vi "CRYAddStep Popup Menu.vi"(9 "Tag":string, 10 "Tree Reference In":refnum<vi>, 11 "Menu Ref In":refnum<k9>) -> (3 "Menu Ref Out":refnum<k9>)   [LabVIEW 2013]
uses:
  CRYMainGlobal.vi
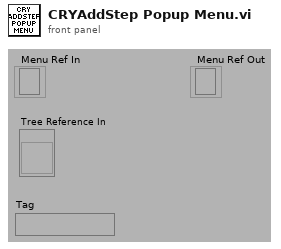
[diagram p1: front panel]
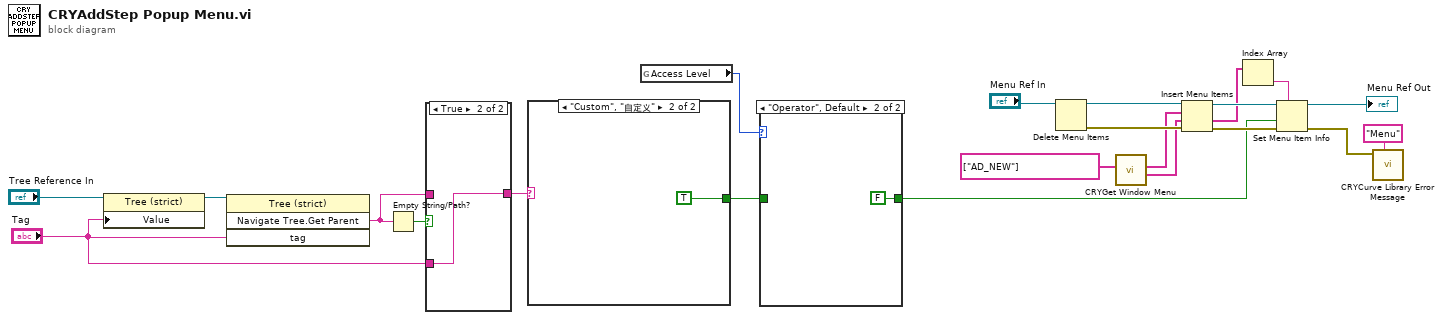
[diagram p0: block diagram]
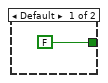
[diagram p3: hidden frame]
diagram:
  n1 = property class="Tree (strict)"(reference="Tree Reference In", "Value"="Tag") -> (reference out=w3:refnum<vi>)  [unwired: 1 in, 1 out]
  n2 = invoke class="Tree (strict)" method="Navigate Tree.Get Parent"(reference=w3, "tag"="Tag") -> ("Navigate Tree:Get Parent"=w15:string)  [unwired: 2 in, 3 out]
  n3 = Empty String/Path?(string/path=w15) -> (empty?=w16:bool)
  n4 = case shown="True" w16 {
    tunnel: w15 -> [w23 _]
    tunnel: [w23 w24] -> w14
    tunnel: "Tag" -> [_ w24]
    frame False {
    }
    frame True {
    }
  }
  n5 = case shown="\"Custom\", \"自定义\"" w14 {
    tunnel: [FALSE ("checked") TRUE ("checked")] -> w5
    frame Default {
    }
    frame "Custom", "自定义" {
    }
  }
  n6 = global read "CRYMainGlobal.vi" "Access Level"() -> (w6:enum16{"Engineer", "Technician", "Operator"})
  n7 = case shown="\"Operator\", Default" w6 {
    tunnel: w5 -> [w27 _]
    tunnel: [w27 FALSE ("checked")] -> w4
    frame "Engineer" {
    }
    frame "Operator", Default {
    }
  }
  n8 = Delete Menu Items(9:"Menu Ref In") -> (0:w19:errorcluster, 3:w20:refnum<k9>)  [unwired: 2 in, 1 out]
  n9 = call "CRYGet Window Menu.vi"("Tags"=string[] ["AD_NEW"] ("item names")) -> ("Tags_Out"=w12:string[], "Names_Out"=w13:string[])  [unwired: 8 in, 1 out]
  n10 = Insert Menu Items(6:w19, 7:w12, 8:w13, 9:w20) -> (0:w9:errorcluster, 1:w8:string[], 3:w10:refnum<k9>)  [unwired: 2 out]
  n11 = Index Array(array=w8) -> (element=w7:string)  [unwired: 1 in]
  n12 = Set Menu Item Info(7:w7, 8:w9, 9:w4, 11:w10) -> (0:w18:errorcluster, 3:→"Menu Ref Out":refnum<k9>)  [unwired: 3 in]
  n13 = call "CRYCurve Library Error Message.vi"("sAction"="Menu", "error IO"=w18) -> ()  [unwired: 10 in]
